vi "Check All Position.vi"(11 "chesses":T1=[[0, 1, 2, 0, 0, 0, 0], [0, 2, 1, 0, 0, 0, 0], [0, 0, 0, 2, 0, 0, 0], [0, 0, 0, 0, 0, 0, 0], [0, 0, 0, 0, 0, 0, 0]]) -> (1 "available white position":i32[][](array[numeric]), 2 "available black position":i32[][](array[numeric]), 4 "available black position number":i32, 6 "available white position number":i32)   [LabVIEW 2018, in "Othello.xctl"]
doc: "本VI是为《我和LabVIEW》一书编写的示例。\n关于本书的介绍请参考网页：\nhttp://ruanqizhen.spaces.live.com/blog/cns!5852D4F797C53FB6!4310.entry"
uses:
  Othello.xctl
  Control/Pict Ring Chess.ctl
  Ability/Data.ctl
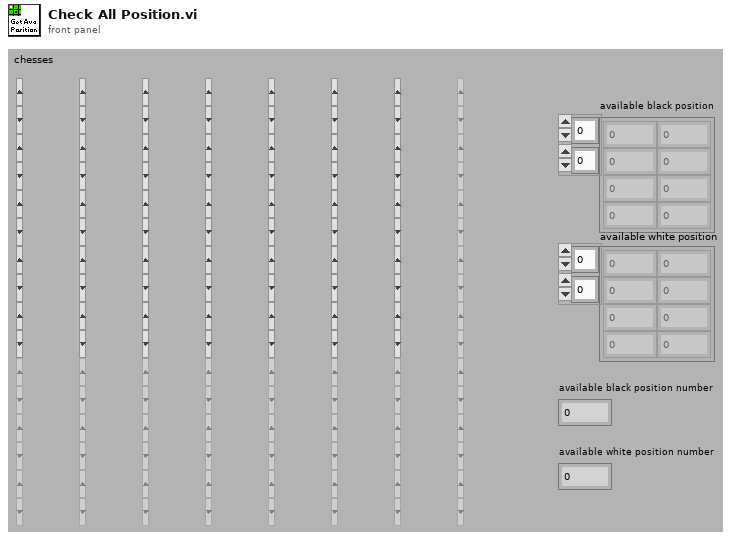
[diagram p1: front panel]
types:
  T1 = typedef "Othello.xctl/Data.ctl" = T2[][]
  T2 = typedef "Othello.xctl/Pict Ring Chess.ctl" = u16
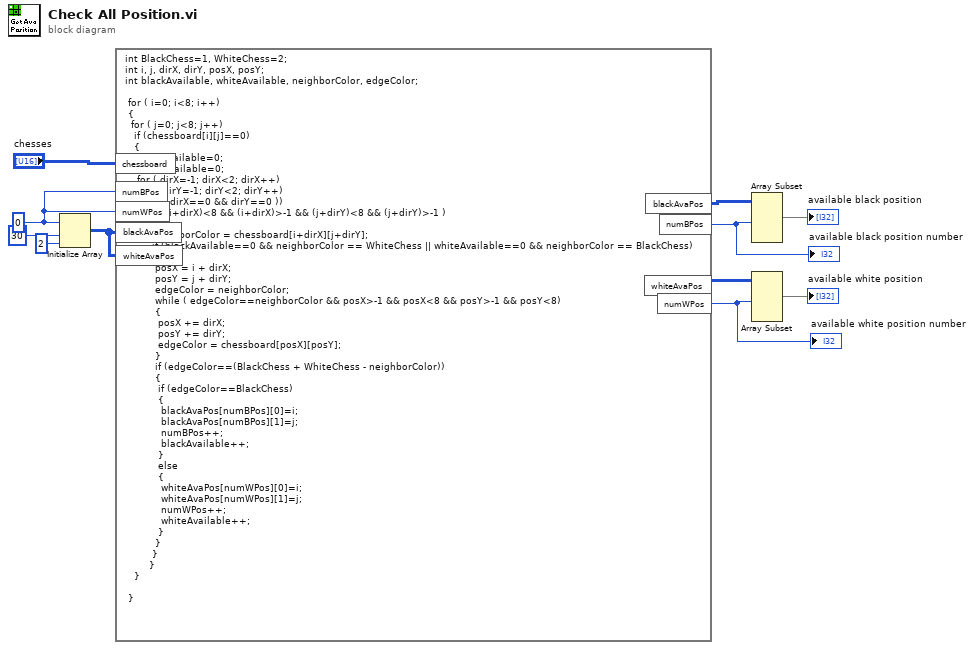
[diagram p0: block diagram]
diagram:
  w8 = 0 ("元素")
  n1 = Initialize Array(w8, 30 ("维数大小"), 2 ("维数大小")) -> (w10:i32[][])
  n2 = formula code="int BlackChess=1, WhiteChess=2;\nint i, j, dirX, dirY, posX, posY;\nint blackAvailable, whiteAvailable, neighborColor, edgeColor;\t\n\n\tfor ( i=0; i<8; i++)\n\t{\n\t\tfor ( j=0; j<8; j++)\n\t\t\tif (chessboard[i][j]==0)\n\t\t\t{\n\t\t\t\tblackAvailable=0;\n\t\t\t\twhiteAvailable=0;\n\t\t\t\tfor ( dirX=-1; dirX<2; dirX++)\n\t\t\t\t\tfor ( dirY=-1; dirY<2; dirY++)\n\t\t\t\t\t\tif ( !( dirX==0 && dirY==0 ))\n\t\t\t\t\t\t\t\tif ( (i+dirX)<8 && (i+dirX)>-1 && (j+dirY)<8 && (j+dirY)>-1 )\n\t\t\t\t\t\t\t\t{\n\t\t\t\t\t\t\t\t\tneighborColor = chessboard[i+dirX][j+dirY];\n\t\t\t\t\t\t\t\t\tif (blackAvailable==0 && neighborColor == WhiteChess || whiteAvailable==0 && neighborColor == BlackChess)\n\t\t\t\t\t\t\t\t\t{\n\t\t\t\t\t\t\t\t\t\tposX = i + dirX;\n\t\t\t\t\t\t\t\t\t\tposY = j + dirY;\n\t\t\t\t\t\t\t\t\t\tedgeColor = neighborColor;\n\t\t\t\t\t\t\t\t\t\twhile ( edgeColor==neighborColor && posX>-1 && posX<8 && posY>-1 && posY<8)\n\t\t\t\t\t\t\t\t\t\t{\n\t\t\t\t\t\t\t\t\t\t\tposX += dirX;\n\t\t\t\t\t\t\t\t\t\t\tposY += dirY;\n\t\t\t\t\t\t\t\t\t\t\tedgeColor = chessboard[posX][posY];\n\t\t\t\t\t\t\t\t\t\t}\n\t\t\t\t\t\t\t\t\t\tif (edgeColor==(BlackChess + WhiteChess - neighborColor))\n\t\t\t\t\t\t\t\t\t\t{\n\t\t\t\t\t\t\t\t\t\t\tif (edgeColor==BlackChess)\n\t\t\t\t\t\t\t\t\t\t\t{\n\t\t\t\t\t\t\t\t\t\t\t\tblackAvaPos[numBPos][0]=i;\n\t\t\t\t\t\t\t\t\t\t\t\tblackAvaPos[numBPos][1]=j;\n\t\t\t\t\t\t\t\t\t\t\t\tnumBPos++;\n\t\t\t\t\t\t\t\t\t\t\t\tblackAvailable++;\n\t\t\t\t\t\t\t\t\t\t\t}\n\t\t\t\t\t\t\t\t\t\t\telse\n\t\t\t\t\t\t\t\t\t\t\t{\n\t\t\t\t\t\t\t\t\t\t\t\twhiteAvaPos[numWPos][0]=i;\n\t\t\t\t\t\t\t\t\t\t\t\twhiteAvaPos[numWPos][1]=j;\n\t\t\t\t\t\t\t\t\t\t\t\tnumWPos++;\n\t\t\t\t\t\t\t\t\t\t\t\twhiteAvailable++;\n\t\t\t\t\t\t\t\t\t\t\t}\n\t\t\t\t\t\t\t\t\t\t}\n\t\t\t\t\t\t\t\t\t}\n\t\t\t\t\t\t\t\t}\n\t\t\t}\n\n\t}"("chessboard"="chesses", "blackAvaPos"=w10, "whiteAvaPos"=w10, "numBPos"=w8, "numWPos"=w8) -> ("blackAvaPos"=w6:i32[][], "numBPos"=w5:i32, "whiteAvaPos"=w2:i32[][], "numWPos"=w1:i32)
  "available black position number" <- w5
  "available white position number" <- w1
  n3 = Array Subset(array=w6, length (row)=w5) -> (→"available black position":i32[][])  [unwired: 3 in]
  n4 = Array Subset(array=w2, length (row)=w1) -> (→"available white position":i32[][])  [unwired: 3 in]
